vi "Main.vi"   [LabVIEW 2020]
uses:
  Libraries/NI DAQ/NI DAQ.lvlib
types:
  T1 = typedef "NI DAQ.lvlib/Broadcast Events--cluster.ctl" = cluster{"Module Did Init":refnum<user-event>, "Status Updated":refnum<user-event>, "Error Reported":refnum<user-event>, "Module Did Stop":refnum<user-event>, "Update Module Execution Status":refnum<user-event>}
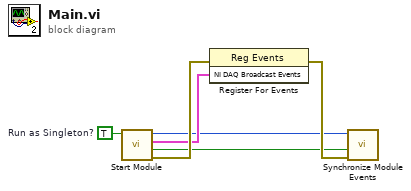
[diagram p0: block diagram]
diagram:
  w6 = TRUE  # Run as Singleton?
  n1 = call "Start Module.vi"("Run as Singleton? (F)"=w6) -> ("error out"=w5:errorcluster, "Wait for Event Sync?"=w2:bool, "NI DAQ Broadcast Events"=w4:T1, "Module ID"=w1:i32)  [unwired: 7 in]
  n2 = register-events(error in=w5, w4) -> (error out=w3:errorcluster)  [unwired: 1 in, 1 out]
  n3 = call "Synchronize Module Events.vi"("error in"=w3, "Wait for Event Sync?"=w2, "Module ID in"=w1) -> ()  [unwired: 7 in, 2 out]
